vi "Create Publish Data Events.vi"(8 "error in (no error)":errorcluster, 11 "UserEvents in":refnum<class "User Events.lvclass">) -> (0 "error out":errorcluster, 3 "UserEvents out":refnum<class "User Events.lvclass">)   [LabVIEW 2016, in "User Events.lvclass"]
uses:
  User Events.lvclass
  User Events.lvclass/User Events.ctl
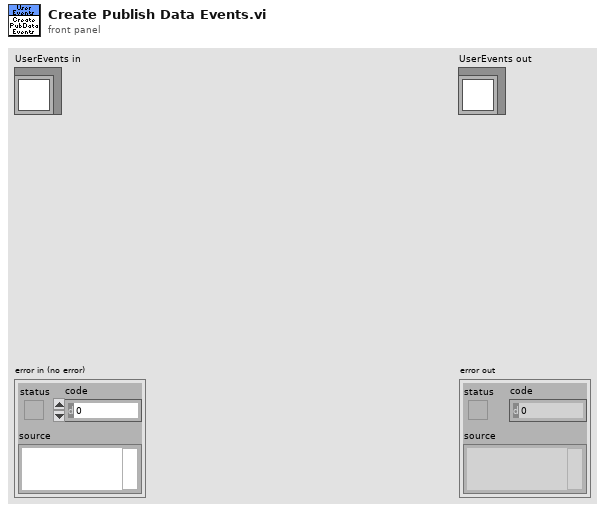
[diagram p1: front panel]
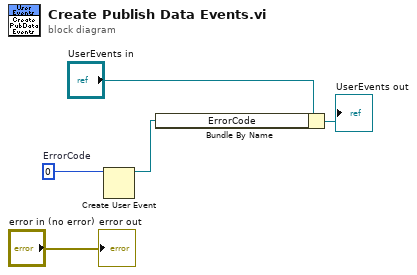
[diagram p0: block diagram]
diagram:
  w2 = 0  # ErrorCode
  n1 = Create User Event(user event datatype=w2) -> (user event=w1:refnum<user-event>)  [unwired: 1 in, 1 out]
  n2 = Bundle By Name(cluster="UserEvents in", "ErrorCode"=w1) -> (→"UserEvents out":refnum<class "User Events.lvclass">)
  "error out" <- "error in (no error)"
